vi "Command (write) - ME.vi"(7 "timeout ms (100)":i32=100, 8 "error in (no error)":errorcluster, 10 "IP":string, 11 "connection ID in":refnum<k16>) -> (0 "error out":errorcluster, 3 "connection ID out":refnum<k16>)   [LabVIEW 2016, in "SMD-7615.lvlib" / "eSCL.lvlib"]
doc: "ME - Motor Enable\nRestores drive current to motor. If the drive cannot be enabled due to the Enable Input (SI) state, the drive will respond with a “&” which indicates that the drive could not be enabled. Enabling the drive also deactivates the Brake Output function (see BO command). Enabling of the motor is delayed by the BD (Brake Disengage) time\ndelay."
uses:
  eSCL.lvlib
  String Command and Param.ctl
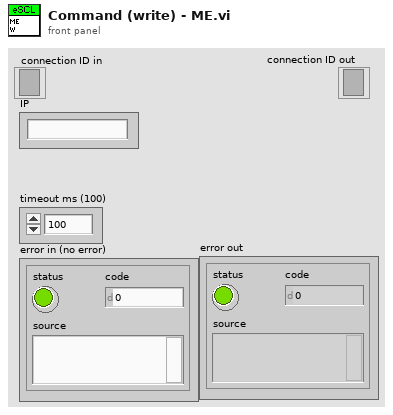
[diagram p1: front panel]
types:
  T1 = typedef "SMD-7615.lvlib/eSCL.lvlib/String Command and Param.ctl" = cluster{"Command":string, "String Parameler":string, "String Parameler Default":string}
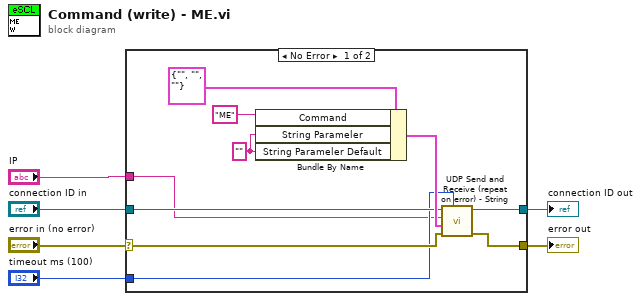
[diagram p0: block diagram]
diagram:
  n1 = case shown="No Error" "error in (no error)" {
    selector: "error in (no error)" -> [w12 w17]
    tunnel: "connection ID in" -> [w10 w18]
    tunnel: [w14 w18] -> w1
    tunnel: [w13 w17] -> w2
    tunnel: "IP" -> [w8 _]
    tunnel: "timeout ms (100)" -> [w9 _]
    frame No Error {
      w7 = "" ("String Parameler Default")
      n2 = Bundle By Name(cluster=T1 {"Command"="", "String Parameler"="", "String Parameler Default"=""} ("String Command & Param"), "Command"="ME", "String Parameler"=w7, "String Parameler Default"=w7) -> (w11:T1)
      n3 = call "UDP Send and Receive (repeat on error) - String.vi"("timeout ms (100)"=w9, "error in (no error)"=w12, "String Command & Param"=w11, "IP"=w8, "connection ID in"=w10) -> ("error out"=w13:errorcluster, "connection ID out"=w14:refnum<k16>)  [unwired: 4 in, 1 out]
    }
    frame Error {
    }
  }
  "connection ID out" <- w1
  "error out" <- w2
